vi "set HTTP header for export.vi"(7 "Content-type (\"application/octet-stream\")":string="application/octet-stream", 10 "filename (\"\")":string, 11 "HTTP Header (\"\")":string) -> (3 "HTTP Header":string)   [LabVIEW 2011]
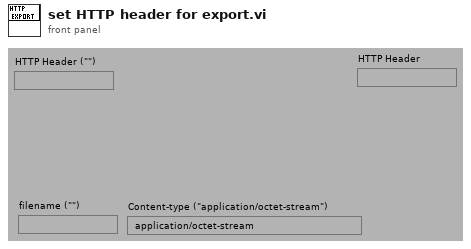
[diagram p1: front panel]
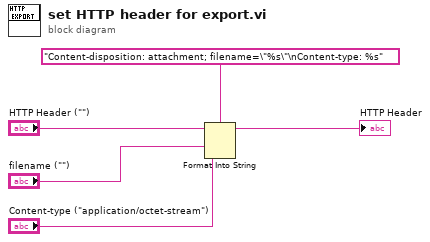
[diagram p0: block diagram]
diagram:
  n1 = Format Into String(format string="Content-disposition: attachment; filename=\"%s\"\nContent-type: %s", initial string="HTTP Header (\"\")", "filename (\"\")", "Content-type (\"application/octet-stream\")") -> (resulting string=→"HTTP Header":string)  [unwired: 1 in, 1 out]
